vi "Main.vi"() -> ()   [LabVIEW 2017]
uses:
  Controllers/Enum_States.ctl
  <vilib>/addons/database/Connection.llb/DB Tools Open Connec (Path).vi
  <vilib>/addons/database/NI_Database_API.lvlib
panel:
  out "PI":bool
  out "zmiana":bool
  out "Stop":bool
  in  "Database User":cluster{"userID":string, "password":string}={"userID"="admin", "password"="admin"}
  out "path":path
  in  "Database":bool
  in  "Szum Button":bool
  in  "Set Point":T1={"T2we Set"=20.0, "V2 Set"=2.0, "T2wy Set"=45.0, "V1 Set"=3.0, "Ki"=1.7999999999999996, "Kp"=1.2} {"Kp" step=0.1; "Ki" step=0.05; "V1 Set" min=0.0 step=0.5; "T2wy Set" step=5.0; "V2 Set" min=0.0 step=0.5; "T2we Set" step=5.0}
  in  "PI_Button":bool
  in  "Clear Chart Button":bool
  out "Twy":cluster{"T1wy":dbl, "T2wy":dbl}
  in  "Parametry 2":T2={"F2 [m^2]"=0.48, "k2 [W/(m^2*K)]"=1175.7, "S2 [m^3]"=5e-05, "c2 [J/(kg*K)]"=4200.0, "p2 [kg/m^3]"=1000.0, "A2 [cm^2]"=3.8}
  in  "Parametry 1":T3={"F1 [m^2]"=0.48, "k1 [W/(m^2*K)]"=1218.4, "S1 [m^3]"=5e-05, "p1 [kg/m^3]"=1000.0, "c1 [J/(kg*K)]"=4200.0, "A1 [cm^2]"=3.8}
  in  "Czynnik Drugi":cluster{"T2we [C]":dbl, "V2 [l/min]":dbl}={"T2we [C]"=20.0, "V2 [l/min]"=3.0} {"V2 [l/min]" min=0.0 step=0.5; "T2we [C]" step=1.0}
  in  "Czynnik Pierwszy":cluster{"V1 [l/min]":dbl, "T1we [C]":dbl}={"V1 [l/min]"=3.0, "T1we [C]"=25.0} {"T1we [C]" step=1.0; "V1 [l/min]" min=0.0 step=0.5}
  out "Rozklad Temperatur":dbl[][](graph)
  out "Przebieg czasowy":cluster{"T1wy":dbl, "T2wy":dbl}(graph)
  in  "Exit_Button":bool
  in  "Stop_Button":bool
  in  "Start_Button":bool
  # "do ukrycia"
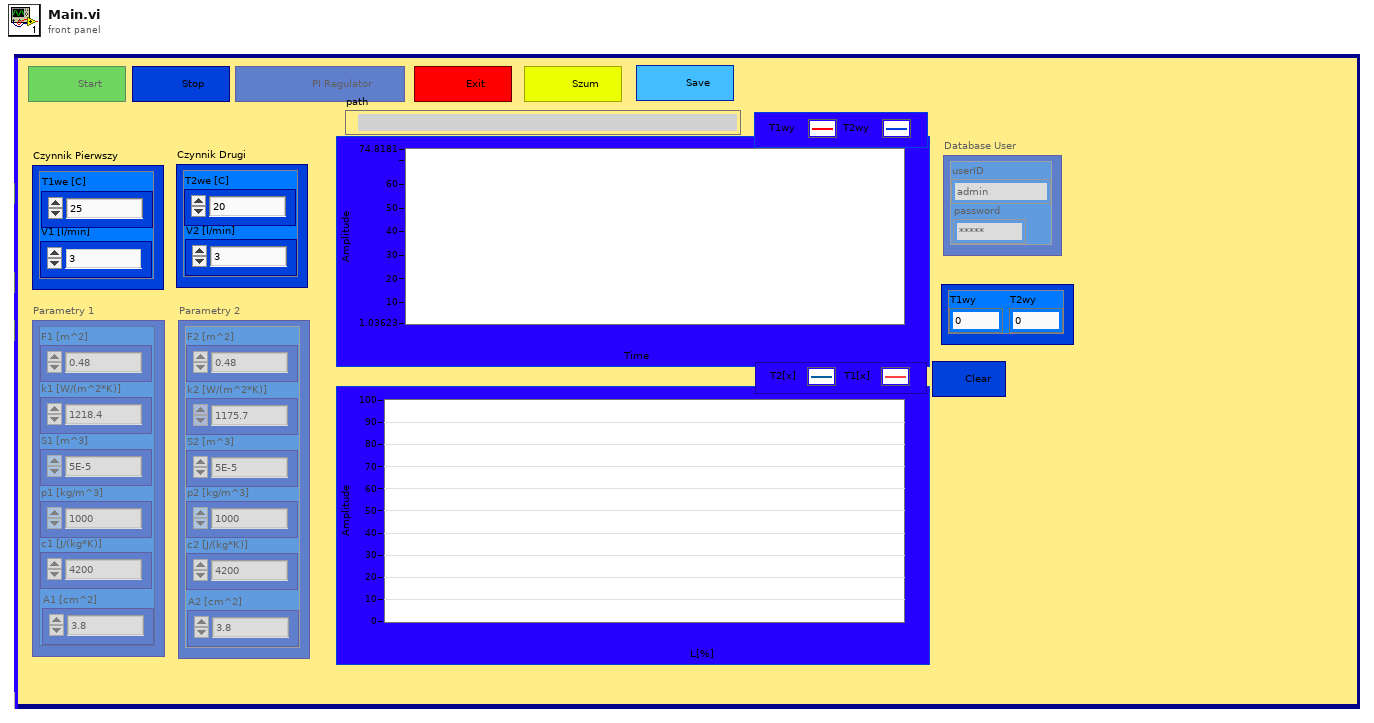
[diagram p1: front panel]
types:
  T1 = cluster{"T2we Set":dbl, "V2 Set":dbl, "T2wy Set":dbl, "V1 Set":dbl, "Ki":dbl, "Kp":dbl}
  T2 = cluster{"F2 [m^2]":dbl, "k2 [W/(m^2*K)]":dbl, "S2 [m^3]":dbl, "c2 [J/(kg*K)]":dbl, "p2 [kg/m^3]":dbl, "A2 [cm^2]":dbl}
  T3 = cluster{"F1 [m^2]":dbl, "k1 [W/(m^2*K)]":dbl, "S1 [m^3]":dbl, "p1 [kg/m^3]":dbl, "c1 [J/(kg*K)]":dbl, "A1 [cm^2]":dbl}
  T4 = enum8{"Enabled", "Disabled", "Disabled and Grayed Out"}
  T5 = typedef "Enum_States.ctl" = enum16{"Initialize", "Exit", "Error", "Run", "Wait"}
  T6 = enum32{"invalid app kind", "Development System", "Run Time System", "Student Edition", "Embedded LabVIEW", "Evaluation", "Custom"}
  T7 = typedef "NI_Database_API.lvlib/Conn ObjectReference.ctl" = refnum<k1>
  T8 = cluster{"w10":dbl, "a1":dbl, "T1we":dbl, "a2":dbl, "w20":dbl, "T2we":dbl, "A1":dbl, "A2":dbl, "V1":dbl, "V2":dbl}
  T9 = cluster{"T1we":dbl, "T2we":dbl, "V1":dbl, "V2":dbl, "Kp":dbl, "Ki":dbl}
  T10 = cluster{"date/time string":string, "T1wy":dbl, "T2wy":dbl, "T1we":dbl, "T2we":dbl, "V1":dbl, "V2":dbl, "Kp":dbl, "Ki":dbl}
  T11 = cluster{"date/time string":string, "F1 [m^2]":dbl, "k1 [W/(m^2*K)]":dbl, "S1 [m^3]":dbl, "p1 [kg/m^3]":dbl, "c1 [J/(kg*K)]":dbl, "A1 [cm^2]":dbl, "F2 [m^2]":dbl, "k2 [W/(m^2*K)]":dbl, "S2 [m^3]":dbl, "c2 [J/(kg*K)]":dbl, "p2 [kg/m^3]":dbl, "A2 [cm^2]":dbl}
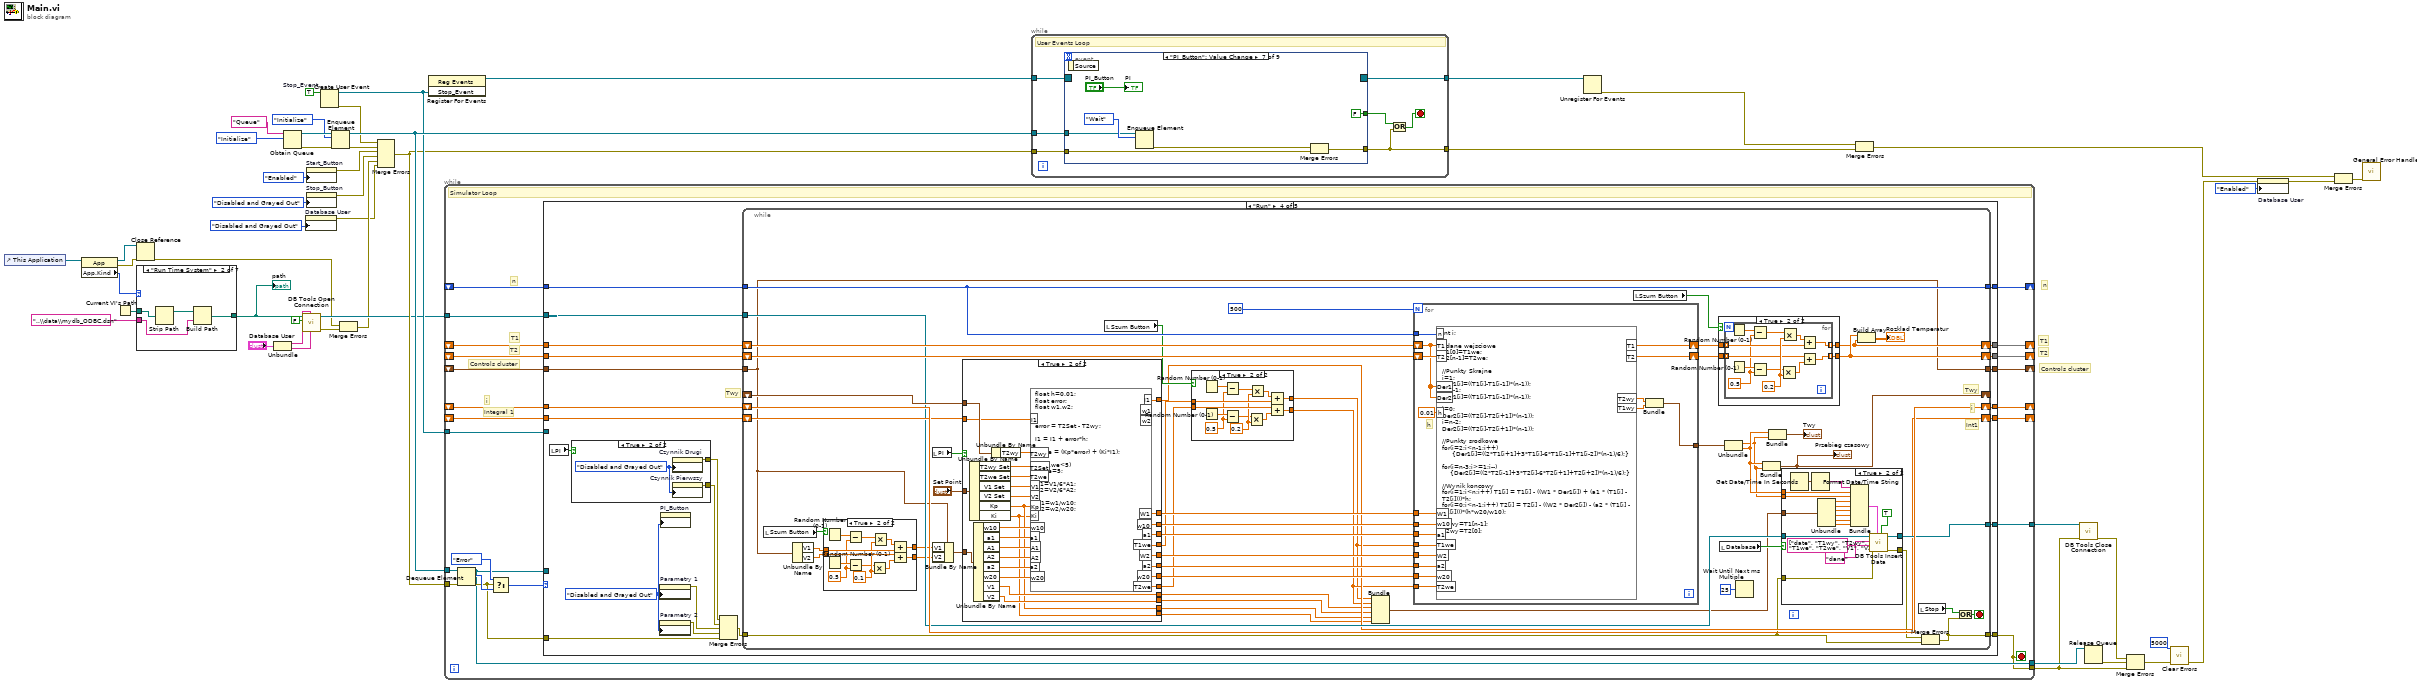
[diagram p0: block diagram]
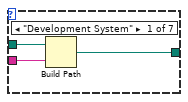
[diagram p2: hidden frame]
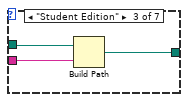
[diagram p3: hidden frame]
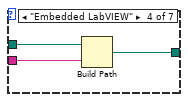
[diagram p4: hidden frame]
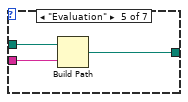
[diagram p5: hidden frame]
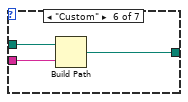
[diagram p6: hidden frame]
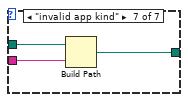
[diagram p7: hidden frame]
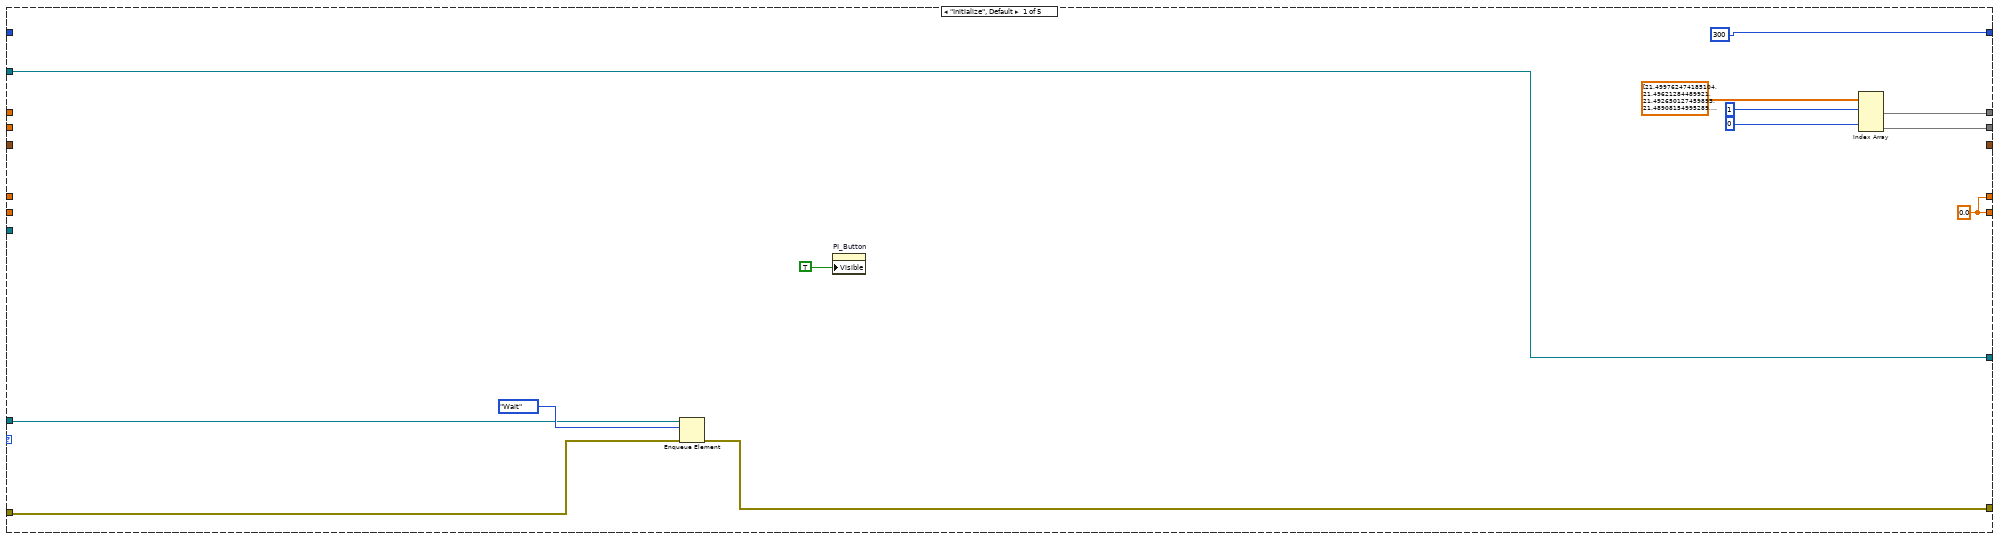
[diagram p8: hidden frame]
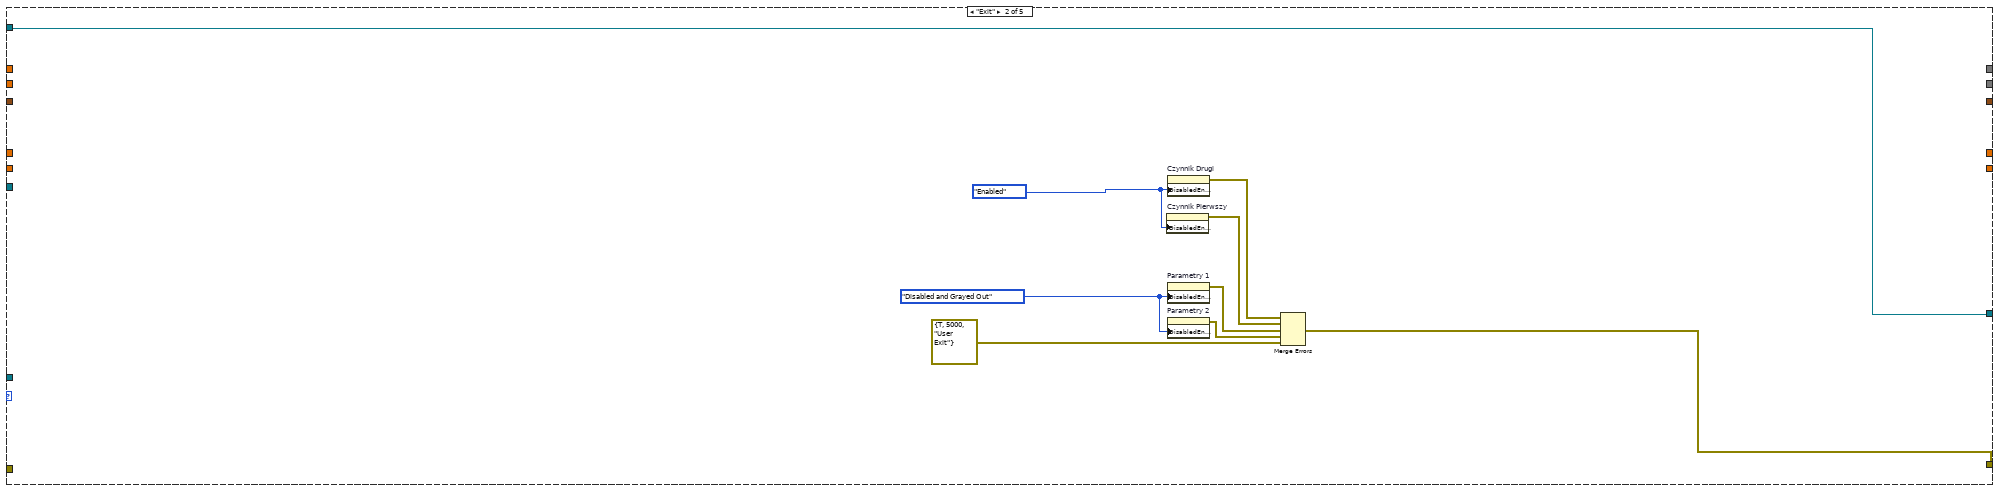
[diagram p9: hidden frame]
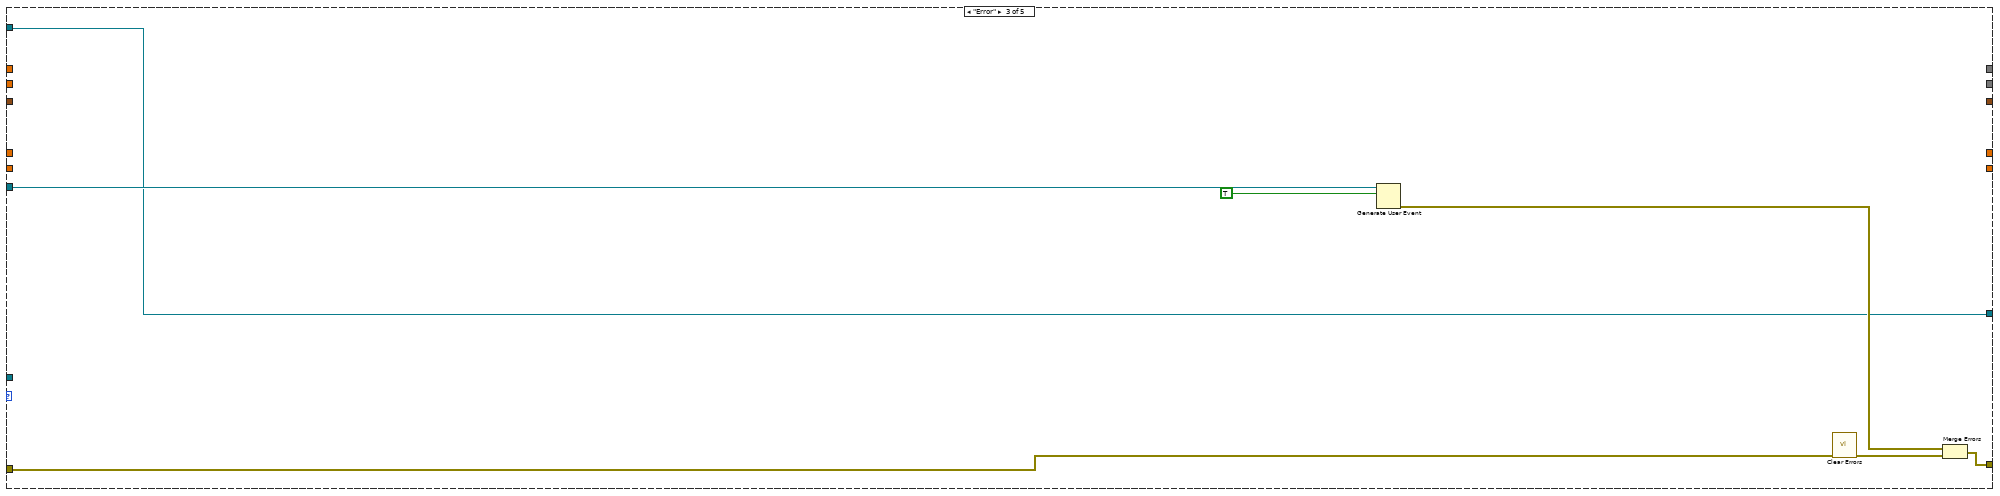
[diagram p10: hidden frame]
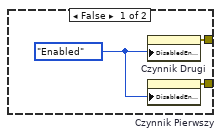
[diagram p11: hidden frame]
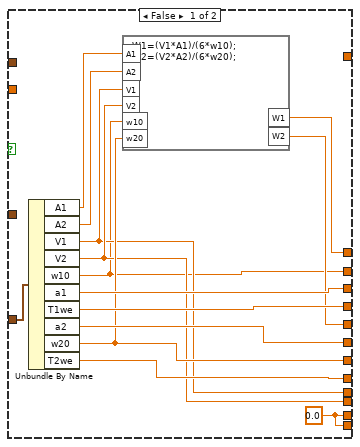
[diagram p15: hidden frame]
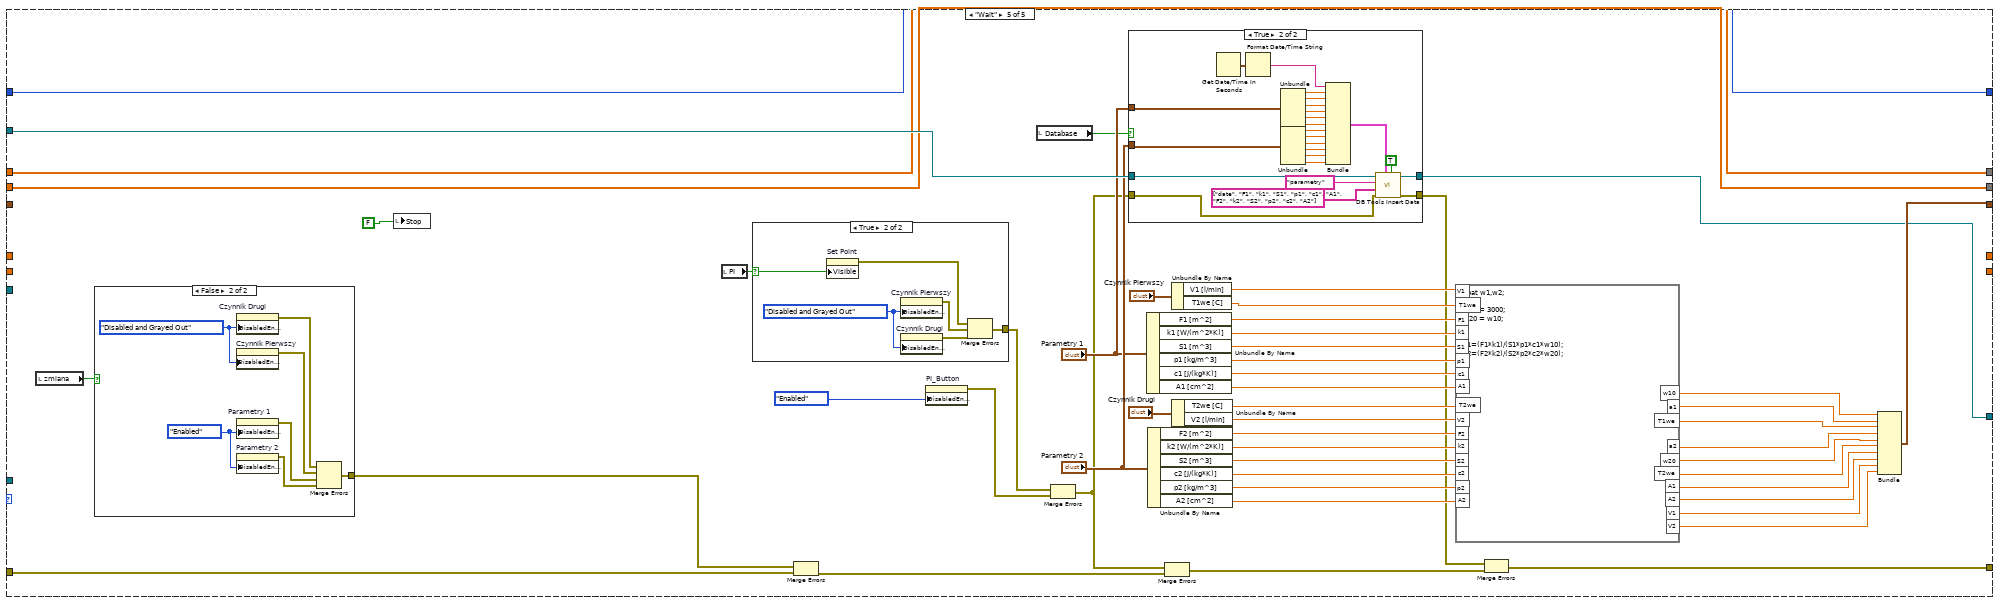
[diagram p17: hidden frame]
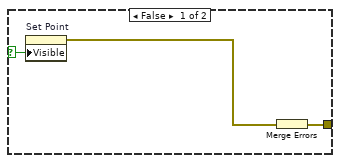
[diagram p19: hidden frame]
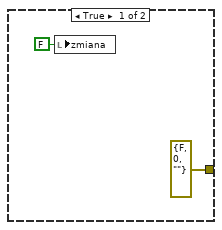
[diagram p20: hidden frame]
diagram:
  w42 = TRUE  # Stop_Event
  # "Controls cluster"
  # "T2"
  # "T1"
  # "n"
  n1 = control-ref of="This Application"() -> (w18:refnum<vi>)
  n2 = property class="App"(reference=w18) -> (reference out=w15:refnum<vi>, error out=w14:errorcluster, "App.Kind"=w17:T6)  [unwired: 1 in]
  n3 = Current VI's Path() -> (path=w16:path)
  n4 = Close Reference(reference=w15, error in (no error)=w14) -> (error out=w11:errorcluster)
  n5 = case shown="\"Run Time System\"" w17 {
    tunnel: [w49 w53 w57 w59 w62 w65 w68] -> w9
    tunnel: w16 -> [w51 w55 w56 w61 w64 w67 w70]
    tunnel: "..\\data\\mydb_ODBC.dsn" -> [w50 w52 w58 w60 w63 w66 w69]
    frame "Development System" {
      n6 = Build Path(base path=w51, name or relative path=w50) -> (appended path=w49:path)
    }
    frame "Run Time System" {
      n7 = Strip Path(path=w55) -> (stripped path=w54:path)  [unwired: 1 out]
      n8 = Build Path(base path=w54, name or relative path=w52) -> (appended path=w53:path)
    }
    frame "Student Edition" {
      n9 = Build Path(base path=w56, name or relative path=w58) -> (appended path=w57:path)
    }
    frame "Embedded LabVIEW" {
      n10 = Build Path(base path=w61, name or relative path=w60) -> (appended path=w59:path)
    }
    frame "Evaluation" {
      n11 = Build Path(base path=w64, name or relative path=w63) -> (appended path=w62:path)
    }
    frame "Custom" {
      n12 = Build Path(base path=w67, name or relative path=w66) -> (appended path=w65:path)
    }
    frame "invalid app kind" {
      n13 = Build Path(base path=w70, name or relative path=w69) -> (appended path=w68:path)
    }
  }
  "path" <- w9
  n14 = Unbundle("Database User") -> ("userID"=w7:string, "password"=w6:string)
  n15 = Obtain Queue(name (unnamed)="Queue", element data type=Enum_States."Initialize") -> (queue out=w46:refnum<queue>, error out=w44:errorcluster)  [unwired: 3 in, 1 out]
  n16 = call-poly <vilib>:"DB Tools Open Connection.vi"("password"=w6, "userID"=w7, "prompt? (F)"=FALSE, "connection information"=w9) -> ("error out"=w13:errorcluster, "connection reference"=w22:T7)  [unwired: 4 in]
  n17 = property on="Database User" class="Clust (strict)"("DisabledEnum"=T4."Disabled and Grayed Out" ("Disabled")) -> (error out=w4:errorcluster)  [unwired: 2 in, 1 out]
  n18 = property on="Start_Button" class="Bool"("DisabledEnum"=T4."Enabled" ("Disabled")) -> (error out=w26:errorcluster)  [unwired: 2 in, 1 out]
  n19 = property on="Stop_Button" class="Bool"("DisabledEnum"=T4."Disabled and Grayed Out" ("Disabled")) -> (error out=w25:errorcluster)  [unwired: 2 in, 1 out]
  n20 = Create User Event(user event datatype=w42) -> (user event=w40:refnum<user-event>, error out=w24:errorcluster)  [unwired: 1 in]
  n21 = Enqueue Element(queue=w46, element=Enum_States."Initialize", error in (no error)=w44) -> (queue out=w45:refnum<queue>, error out=w28:errorcluster)  [unwired: 1 in, 1 out]
  n22 = Merge Errors(w11, w13) -> (w12:errorcluster)
  n23 = Merge Errors(w24, w28, w26, w25, w12, w4) -> (w27:errorcluster)
  n24 = register-events(w40) -> (reference out=w41:refnum<event-registration>)  [unwired: 2 in, 1 out]
  n25 = while {
    tunnel: w45 -> [w93]
    tunnel: w27 -> [w90]
    shift-right: [w88] -> _
    shift-left: _ -> [w79]
    shift-right: [w87] -> _
    shift-left: _ -> [w84]
    shift-right: [w86] -> _
    shift-left: _ -> [w85]
    shift-right: [w83] -> _
    shift-left: _ -> [w82]
    tunnel: w40 -> [w80]
    tunnel: [w72] -> w21
    tunnel: [w81] -> w39
    shift-right: [w78] -> _
    shift-left: _ -> [w75]
    shift-right: [w77] -> _
    shift-left: _ -> [w76]
    tunnel: [w74] -> w23
    tunnel: w22 -> [w73]
    stop <- w72 stop-if-true
    # "i"
    # "Integral 1"
    # "Controls cluster"
    # "T2"
    # "T1"
    # "n"
    # "Simulator Loop"
    n26 = Dequeue Element(queue=w93, error in (no error)=w90) -> (queue out=w81:refnum<queue>, element=w92:T5, error out=w89:errorcluster)  [unwired: 1 in, 1 out]
    n27 = Select(t=Enum_States."Error", s=w89, f=w92) -> (s? t:f=w71:T5)
    n28 = case shown="\"Run\"" w71 {
      tunnel: w89 -> [w105 _ w119 w137 w359]
      tunnel: [300 ("n") _ _ w144 w334] -> w88
      tunnel: w79 -> [_ _ _ w145 w334]
      tunnel: [w102 _ _ w142 w333] -> w87
      tunnel: [w101 _ _ w143 w332] -> w86
      tunnel: w85 -> [_ _ _ w140 w332]
      tunnel: w84 -> [_ _ _ w141 w333]
      tunnel: [_ _ _ w138 w360] -> w83
      tunnel: w82 -> [_ _ _ w139 _]
      tunnel: w81 -> [w103 _ _ _ _]
      tunnel: w80 -> [_ _ w122 _ _]
      tunnel: [w100 _ _ w134 _] -> w78
      tunnel: [w100 _ _ w133 _] -> w77
      tunnel: w76 -> [_ _ _ w132 _]
      tunnel: w75 -> [_ _ _ w131 _]
      tunnel: [w94 w107 w116 w127 w341] -> w74
      tunnel: w73 -> [w94 w107 w116 w126 w342]
      tunnel: [w95 w108 w117 w124 w339] -> w72
      frame "Initialize", Default {
        w100 = 0.0 ("I1")
        n29 = Enqueue Element(queue=w103, element=Enum_States."Wait", error in (no error)=w105) -> (error out=w95:errorcluster)  [unwired: 1 in, 2 out]
        n30 = property on="PI_Button" class="Bool (strict)"("Visible"=TRUE) -> ()  [unwired: 2 in, 2 out]
        n31 = Index Array(array=dbl[][] [[21.499762474185104, 21.49621284489921, 21.492650127459893, 21.48908154995289, 21.48550440911021, 21.481919681710213, 21.478326982335396, 21.474726430005205, 21.471117956921518, 21.467501564412398, 21.463877228158243, 21.46024493328411, 21.456604661365546, 21.452956395239937, 21.449300117224766, 21.445635809777336, 21.44196345525032, 21.43828303598211, 21.434594534263375, 21.43089793234925, 21.427193212454693, 21.423480356756148, 21.41975934739073, 21.416030166456455, 21.41229279601205, 21.40854721807688, 21.404793414630838, 21.40103136761432, 21.3972610589281, 21.393482470433216, 21.389695583950925, 21.385900381262633, 21.382096844109743, 21.378284954193635, 21.37446469317551, 21.37063604267637, 21.366798984276826, 21.362953499517122, 21.359099569896998, 21.355237176875647, 21.351366301871543, 21.347486926262402, 21.343599031385065, 21.33970259853546, 21.33579760896849, 21.331884043897862, 21.327961884496112, 21.324031111894474, 21.32009170718277, 21.31614365140936, 21.312186925581006, 21.30822151066279, 21.304247387578023, 21.300264537208193, 21.29627294039282, 21.292272577929356, 21.288263430573203, 21.284245479037462, 21.280218703992947, 21.27618308606807, 21.27213860584873, 21.268085243878236, 21.264022980657174, 21.2599517966434, 21.25587167225188, 21.2517825878546, 21.24768452378043, 21.243577460315134, 21.23946137770118, 21.235336256137728, 21.2312020757805, 21.227058816741643, 21.222906459089668, 21.218744982849355, 21.214574368001664, 21.210394594483642, 21.206205642188262, 21.20200749096444, 21.197800120616826, 21.19358351090575, 21.189357641547183, 21.185122492212564, 21.180878042528732, 21.176624272077774, 21.17236116039702, 21.168088686978923, 21.16380683127088, 21.1595155726752, 21.15521489054899, 21.150904764204103, 21.146585172906967, 21.142256095878516, 21.137917512294077, 21.133569401283296, 21.12921174192998, 21.124844513272087, 21.120467694301546, 21.11608126396421, 21.111685201159723, 21.107279484741394, 21.10286409351615, 21.098439006244448, 21.094004201640065, 21.089559658370124, 21.085105355054935, 21.08064127026782, 21.076167382535132, 21.071683670336114, 21.067190112102747, 21.06268668621966, 21.058173371024125, 21.05365014480584, 21.049116985806805, 21.04457387222133, 21.04002078219587, 21.03545769382887, 21.030884585170767, 21.026301434223814, 21.02170821894196, 21.0171049172308, 21.012491506947427, 21.00786796590034, 21.003234271849337, 20.998590402505393, 20.993936335530595, 20.989272048537973, 20.98459751909144, 20.979912724705674, 20.97521764284598, 20.970512250928248, 20.965796526318776, 20.96107044633415, 20.956333988241244, 20.951587129256993, 20.946829846548365, 20.942062117232165, 20.93728391837501, 20.93249522699316, 20.927696020052444, 20.922886274468127, 20.918065967104827, 20.913235074776363, 20.90839357424566, 20.903541442224647, 20.898678655374127, 20.893805190303727, 20.888921023571708, 20.884026131684855, 20.879120491098412, 20.874204078215932, 20.869276869389186, 20.86433884091802, 20.859389969050262, 20.854430229981634, 20.849459599855585, 20.84447805476318, 20.839485570743047, 20.83448212378121, 20.82946768981096, 20.824442244712785, 20.819405764314226, 20.81435822438976, 20.80929960066068, 20.804229868794987, 20.79914900440729, 20.794056983058628, 20.78895378025646, 20.78383937145444, 20.77871373205236, 20.773576837395964, 20.768428662776937, 20.7632691834327, 20.758098374546325, 20.752916211246372, 20.747722668606873, 20.742517721647104, 20.7373013453315, 20.73207351456951, 20.726834204215585, 20.72158338906892, 20.716321043873375, 20.711047143317426, 20.70576166203394, 20.700464574600115, 20.695155855537305, 20.689835479310947, 20.68450342033046, 20.67915965294907, 20.673804151463703, 20.668436890114826, 20.6630578430864, 20.657666984505674, 20.652264288443135, 20.646849728912322, 20.641423279869734, 20.63598491521467, 20.630534608789155, 20.62507233437781, 20.619598065707656, 20.614111776448063, 20.608613440210586, 20.603103030548862, 20.597580520958452, 20.592045884876725, 20.586499095682736, 20.580940126697104, 20.57536895118188, 20.569785542340444, 20.564189873317286, 20.558581917197948, 20.552961647008903, 20.547329035717357, 20.541684056231254, 20.536026681398972, 20.53035688400932, 20.52467463679135, 20.518979912414256, 20.513272683487216, 20.507552922559253, 20.501820602119174, 20.496075694595326, 20.490318172355554, 20.484548007707033, 20.478765172896125, 20.47296964010825, 20.467161381467758, 20.461340369037824, 20.455506574820284, 20.44965997075544, 20.44380052872204, 20.437928220537078, 20.432043017955685, 20.426144892670948, 20.420233816313804, 20.414309760452927, 20.408372696594512, 20.402422596182273, 20.39645943059716, 20.39048317115727, 20.38449378911775, 20.37849125567068, 20.37247554194482, 20.366446619005544, 20.36040445785473, 20.354349029430566, 20.34828030460741, 20.34219825419568, 20.336102848941696, 20.329994059527547, 20.323871856570936, 20.317736210625064, 20.3115870921785, 20.305424471654966, 20.299248319413252, 20.29305860574704, 20.28685530088483, 20.280638374989717, 20.2744077981593, 20.268163540425487, 20.261905571754404, 20.255633862046214, 20.249348381135, 20.243049098788603, 20.236735984708467, 20.23040900852951, 20.22406813981997, 20.21771334808124, 20.211344602747765, 20.204961873186868, 20.198565128698633, 20.192154338515657, 20.185729471803004, 20.17929049765806, 20.17283738511035, 20.166370103121356, 20.15988862058441, 20.15339290632452, 20.14688292909826, 20.140358657593595, 20.13382006042971, 20.1272671061569, 20.120699763256376, 20.11411800014012, 20.10752178515079, 20.10091108656152, 20.09428587257573, 20.08764611132706, 20.080991770879056, 20.074322819225547, 20.067639224289234, 20.060940953926355, 20.05422797592062, 20.04750025803777, 20.040757768085356, 20.034000474863543, 20.027228351568695, 20.020441398620374, 20.01363975376117, 20.006824315775056, 20.0], [22.0, 21.99754240534437, 21.99508160726046, 21.992615817584294, 21.990144688811398, 21.987668148203934, 21.985186171871884, 21.982698745872124, 21.980205857773576, 21.97770749552414, 21.975203647077016, 21.972694300381157, 21.970179443357193, 21.967659063901028, 21.965133149881616, 21.96260168914147, 21.96006466949637, 21.957522078735348, 21.95497390462064, 21.952420134887603, 21.949860757244707, 21.94729575937345, 21.944725128928265, 21.942148853536523, 21.939566920798395, 21.936979318286863, 21.934386033547664, 21.93178705409912, 21.929182367432208, 21.92657196101049, 21.923955822269946, 21.921333938619014, 21.918706297438526, 21.916072886081558, 21.91343369187348, 21.91078870211181, 21.90813790406622, 21.90548128497842, 21.90281883206213, 21.900150532503005, 21.897476373458595, 21.89479634205825, 21.892110425403054, 21.88941861056583, 21.886720884590996, 21.884017234494557, 21.881307647264, 21.87859210985827, 21.875870609207684, 21.8731431322139, 21.870409665749868, 21.867670196659642, 21.864924711758434, 21.86217319783255, 21.859415641639274, 21.856652029906826, 21.853882349334327, 21.85110658659169, 21.848324728319568, 21.845536761129345, 21.842742671603013, 21.83994244629304, 21.83713607172246, 21.83432353438471, 21.831504820743596, 21.82867991723324, 21.82584881025794, 21.823011486192186, 21.820167931380592, 21.817318132137824, 21.814462074748466, 21.811599745467014, 21.808731130517817, 21.80585621609494, 21.802974988362244, 21.80008743345319, 21.7971935374708, 21.794293286487626, 21.791386666545634, 21.78847366365617, 21.785554263799884, 21.78262845292666, 21.77969621695557, 21.776757541774792, 21.77381241324151, 21.770860817181884, 21.767902739390994, 21.764938165632728, 21.761967081639728, 21.75898947311336, 21.7560053257236, 21.75301462510895, 21.750017356876448, 21.74701350660155, 21.74400305982803, 21.74098600206797, 21.73796231880166, 21.7349319954775, 21.731895017511995, 21.72885137028962, 21.72580103916281, 21.722744009451855, 21.719680266444808, 21.716609795397464, 21.713532581533293, 21.710448610043294, 21.707357866086017, 21.704260334787413, 21.701156001240793, 21.6980448505068, 21.69492686761325, 21.691802037555153, 21.688670345294558, 21.685531775760534, 21.682386313849104, 21.679233944423128, 21.67607465231224, 21.67290842231281, 21.66973523918785, 21.666555087666943, 21.66336795244617, 21.660173818187992, 21.656972669521256, 21.65376449104108, 21.650549267308772, 21.64732698285178, 21.64409762216359, 21.640861169703683, 21.637617609897433, 21.634366927136014, 21.631109105776396, 21.627844130141213, 21.624571984518695, 21.621292653162595, 21.61800612029213, 21.614712370091887, 21.611411386711758, 21.608103154266853, 21.604787656837416, 21.601464878468793, 21.5981348031713, 21.594797414920183, 21.59145269765553, 21.588100635282192, 21.584741211669666, 21.581374410652124, 21.578000216028208, 21.574618611561064, 21.57122958097821, 21.567833107971463, 21.564429176196807, 21.561017769274386, 21.557598870788436, 21.55417246428716, 21.550738533282654, 21.547297061250845, 21.54384803163142, 21.54039142782774, 21.53692723320671, 21.533455431098776, 21.529976004797795, 21.52648893756097, 21.52299421260878, 21.519491813124866, 21.51598172225602, 21.512463923112, 21.508938398765547, 21.505405132252218, 21.501864106570395, 21.49831530468114, 21.494758709508147, 21.49119430393764, 21.487622070818286, 21.48404199296109, 21.480454053139386, 21.476858234088684, 21.47325451850665, 21.46964288905295, 21.466023328349248, 21.462395818979022, 21.458760343487565, 21.45511688438188, 21.45146542413058, 21.447805945163818, 21.444138429873227, 21.440462860611753, 21.43677921969362, 21.433087489394293, 21.429387651950357, 21.425679689559395, 21.42196358437995, 21.418239318531377, 21.41450687409379, 21.41076623310801, 21.407017377575475, 21.403260289458135, 21.39949495067834, 21.395721343118783, 21.391939448622416, 21.388149248992338, 21.38435072599173, 21.380543861343746, 21.37672863673144, 21.372905033797714, 21.369073034145156, 21.36523261933601, 21.36138377089204, 21.357526470294474, 21.35366069898391, 21.349786438360233, 21.345903669782523, 21.342012374568938, 21.338112533996643, 21.334204129301742, 21.33028714167917, 21.3263615522826, 21.322427342224344, 21.318484492575266, 21.31453298436469, 21.310572798580353, 21.306603916168246, 21.30262631803257, 21.298639985035624, 21.294644897997667, 21.290641037696943, 21.286628384869495, 21.282606920209115, 21.278576624367187, 21.27453747795267, 21.270489461531994, 21.266432555628903, 21.26236674072444, 21.2582919972568, 21.254208305621262, 21.25011564617013, 21.24601399921254, 21.24190334501445, 21.237783663798517, 21.233654935743967, 21.229517140986548, 21.225370259618437, 21.221214271688147, 21.217049157200382, 21.212874896115988, 21.208691468351848, 21.204498853780766, 21.200297032231376, 21.19608598348805, 21.191865687290797, 21.18763612333517, 21.183397271272174, 21.179149110708156, 21.174891621204743, 21.1706247822787, 21.16634857340185, 21.162062974000932, 21.157767963457598, 21.153463521108225, 21.149149626243876, 21.144826258110125, 21.140493395907004, 21.13615101878891, 21.13179910586455, 21.127437636196753, 21.123066588802406, 21.11868594265234, 21.114295676671254, 21.109895769737587, 21.105486200683455, 21.101066948294488, 21.096637991309795, 21.092199308421833, 21.08775087827629, 21.083292679471977, 21.078824690560758, 21.07434689004744, 21.069859256389638, 21.06536176799772, 21.060854403234664, 21.05633714041594, 21.051809957809542, 21.047272833635514, 21.042725746066733, 21.038168673226508, 21.033601593194703, 21.029024483990725, 21.024437323619043, 21.019840089946143, 21.015232761031722, 21.010615314235483, 21.005987728624966, 21.001349978483297, 20.996702050812907, 20.99204389814279, 20.98737556576997, 20.982696848709715, 20.978008216685975, 20.973308320608737, 20.968600717641955, 20.963875750815955]] ("Rozklad Temperatur"), index (row) #1=1 ("index (row)"), index (row) #2=0 ("index (row)")) -> (element #1=w102:dbl[], element #2=w101:dbl[])  [unwired: 2 in]
      }
      frame "Exit" {
        w112 = T4."Disabled and Grayed Out" ("Disabled")
        w113 = T4."Enabled" ("Disabled")
        n32 = property on="Czynnik Pierwszy" class="Clust (strict)"("DisabledEnum"=w113) -> (error out=w110:errorcluster)  [unwired: 2 in, 1 out]
        n33 = property on="Czynnik Drugi" class="Clust (strict)"("DisabledEnum"=w113) -> (error out=w109:errorcluster)  [unwired: 2 in, 1 out]
        n34 = property on="Parametry 1" class="Clust (strict)"("DisabledEnum"=w112) -> (error out=w114:errorcluster)  [unwired: 2 in, 1 out]
        n35 = property on="Parametry 2" class="Clust (strict)"("DisabledEnum"=w112) -> (error out=w115:errorcluster)  [unwired: 2 in, 1 out]
        n36 = Merge Errors(w109, w110, w114, w115, errorcluster {"status"=TRUE, "code"=5000, "source"="User Exit"} ("error constant")) -> (w108:errorcluster)
      }
      frame "Error" {
        n37 = Generate User Event(user event=w122, event data cluster=TRUE ("event data")) -> (error out=w120:errorcluster)  [unwired: 2 in, 1 out]
        n38 = call <vilib>:"Clear Errors.vi"("error in (no error)"=w119) -> ("error out"=w118:errorcluster)  [unwired: 5 in, 1 out]
        n39 = Merge Errors(w120, w118) -> (w117:errorcluster)
      }
      frame "Run" {
        w130 = T4."Disabled and Grayed Out" ("Disabled")
        # "Twy"
        n40 = local read "PI"() -> (w123:bool)
        n41 = case shown="True" w123 {
          tunnel: [w147 w151] -> w129
          tunnel: [w148 w150] -> w128
          frame False {
            w146 = T4."Enabled" ("Disabled")
            n42 = property on="Czynnik Drugi" class="Clust (strict)"("DisabledEnum"=w146) -> (error out=w148:errorcluster)  [unwired: 2 in, 1 out]
            n43 = property on="Czynnik Pierwszy" class="Clust (strict)"("DisabledEnum"=w146) -> (error out=w147:errorcluster)  [unwired: 2 in, 1 out]
          }
          frame True {
            w149 = T4."Disabled and Grayed Out" ("Disabled")
            n44 = property on="Czynnik Drugi" class="Clust (strict)"("DisabledEnum"=w149) -> (error out=w150:errorcluster)  [unwired: 2 in, 1 out]
            n45 = property on="Czynnik Pierwszy" class="Clust (strict)"("DisabledEnum"=w149) -> (error out=w151:errorcluster)  [unwired: 2 in, 1 out]
          }
        }
        n46 = property on="Parametry 1" class="Clust (strict)"("DisabledEnum"=w130) -> (error out=w136:errorcluster)  [unwired: 2 in, 1 out]
        n47 = property on="Parametry 2" class="Clust (strict)"("DisabledEnum"=w130) -> (error out=w135:errorcluster)  [unwired: 2 in, 1 out]
        n48 = property on="PI_Button" class="Bool (strict)"("DisabledEnum"=w130) -> ()  [unwired: 2 in, 2 out]
        n49 = Merge Errors(w128, w129, w136, w135, w137) -> (w125:errorcluster)
        n50 = while {
          tunnel: w145 -> [w202]
          tunnel: [w202] -> w144
          shift-right: [w194] -> w143
          shift-left: w140 -> [w191]
          shift-right: [w193] -> w142
          shift-left: w141 -> [w190]
          tunnel: w139 -> [w161]
          tunnel: [w161] -> w138
          shift-right: [w203] -> w134
          shift-left: w131 -> [w203]
          shift-right: [w198] -> _
          shift-left: _ -> [w200]
          shift-right: [w172] -> w133
          shift-left: w132 -> [w199]
          tunnel: [w177] -> w127
          tunnel: w126 -> [w178]
          tunnel: w125 -> [w165]
          tunnel: [w163] -> w124
          stop <- w179 stop-if-true
          # "i"
          # "Int1"
          # "Twy"
          n51 = local read "Szum Button"() -> (w167:bool)
          n52 = Unbundle By Name(w161) -> ("V1"=w162:dbl, "V2"=w168:dbl)
          n53 = case shown="True" w167 {
            tunnel: w162 -> [w206 w218]
            tunnel: w168 -> [w205 w217]
            tunnel: [w205 w216] -> w169
            tunnel: [w206 w215] -> w170
            frame False {
            }
            frame True {
              w207 = 0.5 ("y")
              w214 = 0.1 ("y")
              n54 = Random Number (0-1)() -> (number: 0 to 1=w211:dbl)
              n55 = Random Number (0-1)() -> (number: 0 to 1=w209:dbl)
              n56 = Subtract(x=w211, y=w207) -> (x-y=w210:dbl)
              n57 = Subtract(x=w209, y=w207) -> (x-y=w208:dbl)
              n58 = Multiply(x=w208, y=w214) -> (x*y=w213:dbl)
              n59 = Multiply(x=w210, y=w214) -> (x*y=w212:dbl)
              n60 = Add(x=w212, y=w218) -> (x+y=w215:dbl)
              n61 = Add(x=w217, y=w213) -> (x+y=w216:dbl)
            }
          }
          n62 = local read "PI"() -> (w183:bool)
          n63 = Bundle By Name(cluster=w161, "V1"=w170, "V2"=w169) -> (w171:T8)
          n64 = case shown="True" w183 {
            tunnel: w171 -> [w284 w312]
            tunnel: [w279 w296] -> w182
            tunnel: [w272 w297] -> w184
            tunnel: [w283 w294] -> w188
            tunnel: [w282 w295] -> w176
            tunnel: [w278 w298] -> w187
            tunnel: [w281 w299] -> w186
            tunnel: [w277 w300] -> w185
            tunnel: [w280 w301] -> w175
            tunnel: w200 -> [_ w307]
            tunnel: w199 -> [_ w292]
            tunnel: [_ w293] -> w172
            tunnel: "Set Point" -> [_ w289]
            tunnel: [w276 w288] -> w155
            tunnel: [w275 w287] -> w156
            tunnel: [w271 w286] -> w154
            tunnel: [w271 w285] -> w153
            frame False {
              w271 = 0.0 ("Kp")
              n65 = Unbundle By Name(w284) -> ("A1"=w274:dbl, "A2"=w273:dbl, "V1"=w275:dbl, "V2"=w276:dbl, "w10"=w272:dbl, "a1"=w283:dbl, "T1we"=w282:dbl, "a2"=w281:dbl, "w20"=w277:dbl, "T2we"=w280:dbl)
              n66 = formula code="W1=(V1*A1)/(6*w10);\nW2=(V2*A2)/(6*w20);"("V1"=w275, "V2"=w276, "A1"=w274, "A2"=w273, "w10"=w272, "w20"=w277) -> ("W1"=w279:dbl, "W2"=w278:dbl)
            }
            frame True {
              n67 = Unbundle By Name(w289) -> ("T2wy Set"=w305:dbl, "T2we Set"=w304:dbl, "V1 Set"=w303:dbl, "V2 Set"=w302:dbl, "Kp"=w286:dbl, "Ki"=w285:dbl)
              n68 = Unbundle By Name(w312) -> ("w10"=w311:dbl, "a1"=w310:dbl, "A1"=w291:dbl, "A2"=w290:dbl, "a2"=w309:dbl, "w20"=w308:dbl, "V1"=w287:dbl, "V2"=w288:dbl)
              n69 = Unbundle By Name(w307) -> ("T2wy"=w306:dbl)
              n70 = formula code="float h=0.01;\nfloat error;\nfloat w1,w2;\n\n\nerror = T2Set - T2wy;\n\nI1 = I1 + error*h;\n\nT1we = (Kp*error) + (Ki*I1);\n\nif (T1we<5)\nT1we=5;\n\nw1=V1/6*A1;\nw2=V2/6*A2;\n\nW1=w1/w10;\nW2=w2/w20;"("w10"=w311, "a1"=w310, "a2"=w309, "w20"=w308, "T2wy"=w306, "T2Set"=w305, "T2we"=w304, "V1"=w303, "V2"=w302, "Kp"=w286, "Ki"=w285, "I1"=w292, "A1"=w291, "A2"=w290) -> ("W1"=w296:dbl, "w10"=w297:dbl, "a1"=w294:dbl, "T1we"=w295:dbl, "W2"=w298:dbl, "a2"=w299:dbl, "w20"=w300:dbl, "T2we"=w301:dbl, "I1"=w293:dbl)  [unwired: 2 out]
            }
          }
          n71 = local read "Szum Button"() -> (w174:bool)
          n72 = case shown="True" w174 {
            tunnel: w176 -> [w241 w253]
            tunnel: w175 -> [w240 w252]
            tunnel: [w240 w251] -> w158
            tunnel: [w241 w250] -> w157
            frame False {
            }
            frame True {
              w242 = 0.5 ("y")
              w249 = 0.2 ("y")
              n73 = Random Number (0-1)() -> (number: 0 to 1=w246:dbl)
              n74 = Random Number (0-1)() -> (number: 0 to 1=w244:dbl)
              n75 = Subtract(x=w246, y=w242) -> (x-y=w245:dbl)
              n76 = Subtract(x=w244, y=w242) -> (x-y=w243:dbl)
              n77 = Multiply(x=w243, y=w249) -> (x*y=w248:dbl)
              n78 = Multiply(x=w245, y=w249) -> (x*y=w247:dbl)
              n79 = Add(x=w247, y=w253) -> (x+y=w250:dbl)
              n80 = Add(x=w252, y=w248) -> (x+y=w251:dbl)
            }
          }
          n81 = Bundle("T1we"=w157, "T2we"=w158, "V1"=w156, "V2"=w155, "Kp"=w154, "Ki"=w153) -> (w152:T9)  [unwired: 1 in]
          n82 = for {
            N: 500 -> [_]
            tunnel: w202 -> [w270]
            tunnel: [w267] -> w192
            tunnel: w188 -> [w264]
            tunnel: w157 -> [w263]
            tunnel: w187 -> [w262]
            tunnel: w186 -> [w261]
            tunnel: w185 -> [w260]
            tunnel: w158 -> [w259]
            tunnel: w184 -> [w254]
            tunnel: w182 -> [w258]
            shift-right: [w268] -> w195
            shift-left: w191 -> [w266]
            shift-right: [w269] -> w196
            shift-left: w190 -> [w265]
            # "h"
            n83 = formula code="int i;\n\n//dane wejsciowe\nT1[0]=T1we;\nT2[n-1]=T2we;\n\n//Punkty Skrajne\ni=1;\nDer1[i]=((T1[i]-T1[i-1])*(n-1));\ni=n-1;\nDer1[i]=((T1[i]-T1[i-1])*(n-1));\n\ni=0;\nDer2[i]=((T2[i]-T2[i+1])*(n-1));\ni=n-2;\nDer2[i]=((T2[i]-T2[i+1])*(n-1));\n\n//Punkty srodkowe\nfor(i=2;i<n-1;i++)\n     {Der1[i]=((2*T1[i+1]+3*T1[i]-6*T1[i-1]+T1[i-2])*(n-1)/6);}\n\nfor(i=n-3;i>=1;i--)\n    {Der2[i]=((2*T2[i-1]+3*T2[i]-6*T2[i+1]+T2[i+2])*(n-1)/6);}\n\n//Wynik koncowy\nfor(i=1;i<n;i++) T1[i] = T1[i] - ((W1 * Der1[i]) + (a1 * (T1[i] - T2[i])))*h;\nfor(i=0;i<n-1;i++) T2[i] = T2[i] - ((W2 * Der2[i]) - (a2 * (T1[i] - T2[i])))*(h*w20/w10);\n\nT1wy=T1[n-1];\nT2wy=T2[0];"("W1"=w258, "w10"=w254, "a1"=w264, "T1we"=w263, "W2"=w262, "a2"=w261, "w20"=w260, "T2we"=w259, "n"=w270, "T1"=w265, "T2"=w266, "Der1"=w265, "Der2"=w265, "h"=0.01) -> ("T1"=w269:dbl[], "T2"=w268:dbl[], "T1wy"=w256:dbl, "T2wy"=w255:dbl)
            n84 = Bundle("T2wy"=w255, "T1wy"=w256) -> (w267:cluster{"T2wy":dbl, "T1wy":dbl})  [unwired: 1 in]
          }
          n85 = local read "Szum Button"() -> (w166:bool)
          n86 = case shown="True" w166 {
            tunnel: w196 -> [w314 w318]
            tunnel: w195 -> [w313 w317]
            tunnel: [w313 w316] -> w194
            tunnel: [w314 w315] -> w193
            frame False {
            }
            frame True {
              n87 = for {
                tunnel: w318 -> [w326] mode=indexing
                tunnel: w317 -> [w329] mode=indexing
                tunnel: [w325] -> w316 mode=indexing
                tunnel: [w324] -> w315 mode=indexing
                w319 = 0.5 ("y")
                w330 = 0.2 ("y")
                n88 = Random Number (0-1)() -> (number: 0 to 1=w323:dbl)
                n89 = Random Number (0-1)() -> (number: 0 to 1=w321:dbl)
                n90 = Subtract(x=w323, y=w319) -> (x-y=w322:dbl)
                n91 = Subtract(x=w321, y=w319) -> (x-y=w320:dbl)
                n92 = Multiply(x=w320, y=w330) -> (x*y=w328:dbl)
                n93 = Multiply(x=w322, y=w330) -> (x*y=w327:dbl)
                n94 = Add(x=w327, y=w326) -> (x+y=w324:dbl)
                n95 = Add(x=w329, y=w328) -> (x+y=w325:dbl)
              }
            }
          }
          n96 = local read "Database"() -> (w173:bool)
          n97 = Unbundle(w192) -> ("T2wy"=w159:dbl, "T1wy"=w160:dbl)
          n98 = Wait Until Next ms Multiple(millisecond multiple=u32 25) -> ()  [unwired: 1 out]
          n99 = Bundle("T1wy"=w160, "T2wy"=w159) -> (w198:cluster{"T1wy":dbl, "T2wy":dbl})  [unwired: 1 in]
          "Przebieg czasowy" <- w198
          n100 = Bundle("T1wy"=w160, "T2wy"=w159) -> (→"Twy":cluster{"T1wy":dbl, "T2wy":dbl})  [unwired: 1 in]
          n101 = case shown="True" w173 {
            tunnel: w178 -> [w220 w239]
            tunnel: [w220 w238] -> w177
            tunnel: w165 -> [w219 w232]
            tunnel: [w219 w231] -> w164
            tunnel: w160 -> [_ w230]
            tunnel: w159 -> [_ w229]
            tunnel: w152 -> [_ w228]
            frame False {
            }
            frame True {
              n102 = Get Date/Time In Seconds() -> (seconds since 1Jan1904=w236:timestamp)
              n103 = Format Date/Time String(seconds (now)=w236) -> (date/time string=w235:string)  [unwired: 2 in]
              n104 = Unbundle(w228) -> ("T1we"=w227:dbl, "T2we"=w226:dbl, "V1"=w225:dbl, "V2"=w224:dbl, "Kp"=w223:dbl, "Ki"=w222:dbl)
              n105 = Bundle("date/time string"=w235, "T1wy"=w230, "T2wy"=w229, "T1we"=w227, "T2we"=w226, "V1"=w225, "V2"=w224, "Kp"=w223, "Ki"=w222) -> (w234:T10)  [unwired: 1 in]
              n106 = call <vilib>:"DB Tools Insert Data.vi"("create table? (F)"=TRUE, "data"=w234, "error in (no error)"=w232, "columns"=string[] ["date", "T1wy", "T2wy", "T1we", "T2we", "V1", "V2", "KP", "KI"], "table"="dane", "connection reference"=w239) -> ("error out"=w231:errorcluster, "connection reference out"=w238:T7)  [unwired: 4 in]
            }
          }
          n107 = Build Array(w194, w193) -> (→"Rozklad Temperatur":dbl[][])
          n108 = local read "Stop"() -> (w180:bool)
          n109 = Merge Errors(w164, w165) -> (w163:errorcluster)
          n110 = Or(x=w180, y=w163) -> (x .or. y?=w179:bool)
        }
      }
      frame "Wait" {
        n111 = local read "zmiana"() -> (w355:bool)
        n112 = case shown="False" w355 {
          tunnel: [errorcluster {"status"=FALSE, "code"=0, "source"=""} ("error IO") w421] -> w354
          frame True {
            n113 = local write "zmiana"(FALSE ("zmiana")) -> ()
          }
          frame False {
            w420 = T4."Enabled" ("Disabled")
            w424 = T4."Disabled and Grayed Out" ("Disabled")
            n114 = property on="Czynnik Pierwszy" class="Clust (strict)"("DisabledEnum"=w424) -> (error out=w419:errorcluster)  [unwired: 2 in, 1 out]
            n115 = property on="Czynnik Drugi" class="Clust (strict)"("DisabledEnum"=w424) -> (error out=w418:errorcluster)  [unwired: 2 in, 1 out]
            n116 = property on="Parametry 1" class="Clust (strict)"("DisabledEnum"=w420) -> (error out=w422:errorcluster)  [unwired: 2 in, 1 out]
            n117 = property on="Parametry 2" class="Clust (strict)"("DisabledEnum"=w420) -> (error out=w423:errorcluster)  [unwired: 2 in, 1 out]
            n118 = Merge Errors(w418, w419, w422, w423) -> (w421:errorcluster)
          }
        }
        n119 = local write "Stop"(FALSE ("Stop_Led")) -> ()
        n120 = local read "PI"() -> (w352:bool)
        n121 = case shown="True" w352 {
          selector: w352 -> [w409 w415]
          tunnel: [w407 w412] -> w351
          frame False {
            n122 = property on="Set Point" class="Clust (strict)"("Visible"=w409) -> (error out=w408:errorcluster)  [unwired: 2 in, 1 out]
            n123 = Merge Errors(w408) -> (w407:errorcluster)
          }
          frame True {
            w414 = T4."Disabled and Grayed Out" ("Disabled")
            n124 = property on="Set Point" class="Clust (strict)"("Visible"=w415) -> (error out=w410:errorcluster)  [unwired: 2 in, 1 out]
            n125 = property on="Czynnik Pierwszy" class="Clust (strict)"("DisabledEnum"=w414) -> (error out=w411:errorcluster)  [unwired: 2 in, 1 out]
            n126 = property on="Czynnik Drugi" class="Clust (strict)"("DisabledEnum"=w414) -> (error out=w413:errorcluster)  [unwired: 2 in, 1 out]
            n127 = Merge Errors(w410, w411, w413) -> (w412:errorcluster)
          }
        }
        n128 = Merge Errors(w354, w359) -> (w357:errorcluster)
        n129 = property on="PI_Button" class="Bool (strict)"("DisabledEnum"=T4."Enabled" ("Disabled")) -> (error out=w353:errorcluster)  [unwired: 2 in, 1 out]
        n130 = local read "Database"() -> (w331:bool)
        n131 = Merge Errors(w351, w353) -> (w335:errorcluster)
        n132 = case shown="True" w331 {
          tunnel: w342 -> [w381 w406]
          tunnel: [w381 w405] -> w341
          tunnel: [w382 w402] -> w338
          tunnel: "Parametry 2" -> [_ w398]
          tunnel: "Parametry 1" -> [_ w397]
          tunnel: w335 -> [w382 w399]
          frame False {
          }
          frame True {
            n133 = Get Date/Time In Seconds() -> (seconds since 1Jan1904=w401:timestamp)
            n134 = Format Date/Time String(seconds (now)=w401) -> (date/time string=w384:string)  [unwired: 2 in]
            n135 = Unbundle(w397) -> ("F1 [m^2]"=w385:dbl, "k1 [W/(m^2*K)]"=w386:dbl, "S1 [m^3]"=w387:dbl, "p1 [kg/m^3]"=w388:dbl, "c1 [J/(kg*K)]"=w389:dbl, "A1 [cm^2]"=w390:dbl)
            n136 = Unbundle(w398) -> ("F2 [m^2]"=w391:dbl, "k2 [W/(m^2*K)]"=w392:dbl, "S2 [m^3]"=w393:dbl, "c2 [J/(kg*K)]"=w394:dbl, "p2 [kg/m^3]"=w395:dbl, "A2 [cm^2]"=w396:dbl)
            n137 = Bundle("date/time string"=w384, "F1 [m^2]"=w385, "k1 [W/(m^2*K)]"=w386, "S1 [m^3]"=w387, "p1 [kg/m^3]"=w388, "c1 [J/(kg*K)]"=w389, "A1 [cm^2]"=w390, "F2 [m^2]"=w391, "k2 [W/(m^2*K)]"=w392, "S2 [m^3]"=w393, "c2 [J/(kg*K)]"=w394, "p2 [kg/m^3]"=w395, "A2 [cm^2]"=w396) -> (w400:T11)  [unwired: 1 in]
            n138 = call <vilib>:"DB Tools Insert Data.vi"("create table? (F)"=TRUE, "data"=w400, "error in (no error)"=w399, "columns"=string[] ["date", "F1", "k1", "S1", "p1", "c1", "A1", "F2", "k2", "S2", "p2", "c2", "A2"], "table"="parametry", "connection reference"=w406) -> ("error out"=w402:errorcluster, "connection reference out"=w405:T7)  [unwired: 4 in]
          }
        }
        n139 = Unbundle By Name("Parametry 1") -> ("F1 [m^2]"=w368:dbl, "k1 [W/(m^2*K)]"=w367:dbl, "S1 [m^3]"=w366:dbl, "p1 [kg/m^3]"=w365:dbl, "c1 [J/(kg*K)]"=w364:dbl, "A1 [cm^2]"=w363:dbl)
        n140 = Unbundle By Name("Parametry 2") -> ("F2 [m^2]"=w370:dbl, "k2 [W/(m^2*K)]"=w371:dbl, "S2 [m^3]"=w372:dbl, "c2 [J/(kg*K)]"=w373:dbl, "p2 [kg/m^3]"=w374:dbl, "A2 [cm^2]"=w375:dbl)
        n141 = Merge Errors(w335, w357) -> (w340:errorcluster)
        n142 = Unbundle By Name("Czynnik Pierwszy") -> ("V1 [l/min]"=w346:dbl, "T1we [C]"=w377:dbl)
        n143 = Unbundle By Name("Czynnik Drugi") -> ("T2we [C]"=w369:dbl, "V2 [l/min]"=w347:dbl)
        n144 = formula code="float w1,w2;\n\nw10 = 3000;\nw20 = w10;\n\n\na1=(F1*k1)/(S1*p1*c1*w10);\na2=(F2*k2)/(S2*p2*c2*w20);"("F1"=w368, "F2"=w370, "k1"=w367, "k2"=w371, "S1"=w366, "S2"=w372, "c1"=w364, "c2"=w373, "p1"=w365, "p2"=w374, "V1"=w346, "T1we"=w377, "V2"=w347, "T2we"=w369, "A2"=w375, "A1"=w363) -> ("w10"=w343:dbl, "a1"=w344:dbl, "T1we"=w345:dbl, "a2"=w358:dbl, "w20"=w379:dbl, "T2we"=w378:dbl, "A1"=w362:dbl, "A2"=w361:dbl, "V1"=w349:dbl, "V2"=w348:dbl)
        n145 = Merge Errors(w338, w340) -> (w339:errorcluster)
        n146 = Bundle("w10"=w343, "a1"=w344, "T1we"=w345, "a2"=w358, "w20"=w379, "T2we"=w378, "A1"=w362, "A2"=w361, "V1"=w349, "V2"=w348) -> (w360:T8)  [unwired: 1 in]
      }
    }
  }
  n147 = while {
    tunnel: w45 -> [w431]
    tunnel: w41 -> [w430]
    tunnel: w27 -> [w429]
    tunnel: [w426] -> w35
    tunnel: [w428] -> w37
    stop <- w425 stop-if-true
    # "User Events Loop"
    n148 = event shown="[6] \"PI_Button\": Value Change" {
      selector: w430 -> [_ _ _ _ _ _ _ _ _]
      dyn-events: [_ _ _ _ _ _ _ _ _] -> w428
      timeout: _ -> [_ _ _ _ _ _ _ _ _]
      tunnel: w431 -> [w438 w444 _ _ _ w469 w471 w485 w497]
      tunnel: [TRUE w439 FALSE FALSE FALSE FALSE FALSE FALSE FALSE] -> w427
      tunnel: w429 -> [w433 w441 w446 w454 w458 w461 w475 w484 w494]
      tunnel: [w432 w440 w448 w454 w458 w463 w474 w483 w493] -> w426
      event "Exit_Button": Value Change; User Event {
        n149 = event-data() -> ()  [unwired: 1 in, 1 out]
        n150 = Enqueue Element(queue=w438, element=Enum_States."Exit") -> (error out=w434:errorcluster)  [unwired: 2 in, 2 out]
        n151 = local write "Stop"(TRUE ("Stop_Led")) -> ()
        n152 = Merge Errors(w434, w433) -> (w432:errorcluster)
      }
      event Panel Close? {
        w439 = TRUE
        n153 = event-data() -> ()  [unwired: 1 in, 1 out]
        n154 = Enqueue Element(queue=w444, element=Enum_States."Exit") -> (error out=w442:errorcluster)  [unwired: 2 in, 2 out]
        n155 = event-data("Discard?"=w439) -> ()  [unwired: 1 in, 1 out]
        n156 = local write "Stop"(w439) -> ()
        n157 = Merge Errors(w442, w441) -> (w440:errorcluster)
      }
      event "Clear Chart Button": Value Change {
        n158 = event-data() -> ()  [unwired: 1 in, 1 out]
        n159 = case shown="True" "Clear Chart Button" {
          tunnel: [errorcluster {"status"=FALSE, "code"=0, "source"=""} ("error IO") w451] -> w447
          frame False {
          }
          frame True {
            n160 = property on="Przebieg czasowy" class="WFChart (strict)"("History Data"=cluster{"T1wy":dbl, "T2wy":dbl}[] []) -> (error out=w451:errorcluster)  [unwired: 2 in, 1 out]
          }
        }
        n161 = Merge Errors(w447, w446) -> (w448:errorcluster)
      }
      event "Szum Button": Value Change {
        n162 = event-data() -> ()  [unwired: 1 in, 6 out]
        n163 = local write "Szum Button"("Szum Button") -> ()
      }
      event "Database": Value Change {
        n164 = event-data() -> ()  [unwired: 1 in, 6 out]
        n165 = local write "Database"("Database") -> ()
      }
      event "Czynnik Pierwszy", "Czynnik Drugi": Value Change {
        n166 = event-data() -> ()  [unwired: 1 in, 1 out]
        n167 = Enqueue Element(queue=w469, element=Enum_States."Wait") -> (queue out=w467:refnum<queue>, error out=w460:errorcluster)  [unwired: 2 in, 1 out]
        n168 = Enqueue Element(queue=w467, element=Enum_States."Run") -> (error out=w464:errorcluster)  [unwired: 2 in, 2 out]
        n169 = Merge Errors(w464, w460, w461) -> (w463:errorcluster)
        "Stop" <- TRUE ("Stop")
        "zmiana" <- TRUE ("zmiana")
      }
      event "PI_Button": Value Change {
        n170 = event-data() -> ()  [unwired: 1 in, 1 out]
        n171 = Enqueue Element(queue=w471, element=Enum_States."Wait") -> (error out=w470:errorcluster)  [unwired: 2 in, 2 out]
        n172 = Merge Errors(w470, w475) -> (w474:errorcluster)
        "PI" <- "PI_Button"
      }
      event "Start_Button": Value Change {
        n173 = event-data() -> ()  [unwired: 1 in, 1 out]
        n174 = Enqueue Element(queue=w485, element=Enum_States."Run") -> (error out=w479:errorcluster)  [unwired: 2 in, 2 out]
        n175 = property on="Start_Button" class="Bool"("DisabledEnum"=T4."Disabled and Grayed Out" ("Disabled")) -> (error out=w478:errorcluster)  [unwired: 2 in, 1 out]
        n176 = property on="Stop_Button" class="Bool"("DisabledEnum"=T4."Enabled" ("Disabled")) -> (error out=w477:errorcluster)  [unwired: 2 in, 1 out]
        n177 = Merge Errors(w479, w478, w477, w484) -> (w483:errorcluster)
      }
      event "Stop_Button": Value Change {
        n178 = event-data() -> ()  [unwired: 1 in, 1 out]
        n179 = Enqueue Element(queue=w497, element=Enum_States."Wait") -> (error out=w491:errorcluster)  [unwired: 2 in, 2 out]
        n180 = property on="Start_Button" class="Bool"("DisabledEnum"=T4."Enabled" ("Disabled")) -> (error out=w487:errorcluster)  [unwired: 2 in, 1 out]
        n181 = property on="Stop_Button" class="Bool"("DisabledEnum"=T4."Disabled and Grayed Out" ("Disabled")) -> (error out=w488:errorcluster)  [unwired: 2 in, 1 out]
        n182 = local write "Stop"(TRUE ("Stop_Led")) -> ()
        n183 = Merge Errors(w491, w487, w488, w494) -> (w493:errorcluster)
      }
    }
    n184 = Or(x=w427, y=w426) -> (x .or. y?=w425:bool)
  }
  n185 = Unregister For Events(event registration refnum=w37) -> (error out=w36:errorcluster)  [unwired: 1 in]
  n186 = Merge Errors(w36, w35) -> (w34:errorcluster)
  n187 = call <vilib>:"DB Tools Close Connection.vi"("error in (no error)"=w21, "connection reference"=w23) -> ("error out"=w20:errorcluster)  [unwired: 5 in]
  n188 = Release Queue(queue=w39) -> (error out=w38:errorcluster)  [unwired: 2 in, 2 out]
  n189 = Merge Errors(w20, w38, w21) -> (w32:errorcluster)
  n190 = call <vilib>:"Clear Errors.vi"("error in (no error)"=w32, "specific error code to clear (0: all)"=5000) -> ("error out"=w2:errorcluster)  [unwired: 4 in, 1 out]
  n191 = property on="Database User" class="Clust (strict)"(error in=w2, "DisabledEnum"=T4."Enabled" ("Disabled")) -> (error out=w1:errorcluster)  [unwired: 1 in, 1 out]
  n192 = Merge Errors(w34, w1) -> (w33:errorcluster)
  n193 = call <vilib>:"General Error Handler.vi"("error in (no error)"=w33) -> ()  [unwired: 10 in, 5 out]
